vi "PC_RealTimeHardwareDetection.vi"() -> ()   [LabVIEW 2010]
uses:
  <vilib>/nisyscfg/Initialize (Control).vi
  <vilib>/nisyscfg/Close (System).vi
  <vilib>/nisyscfg/Close (Hardware).vi
  C:/Program Files (x86)/National Instruments/LabVIEW 2010/resource/objmgr/nisysapi.rc
  <vilib>/nisyscfg/nisyscfg.lvlib
panel:
  out "Experts":T1(array[cluster])
  in  "Target (localhost)":refnum<k21>="localhost"
  out "Results":string[][](table)
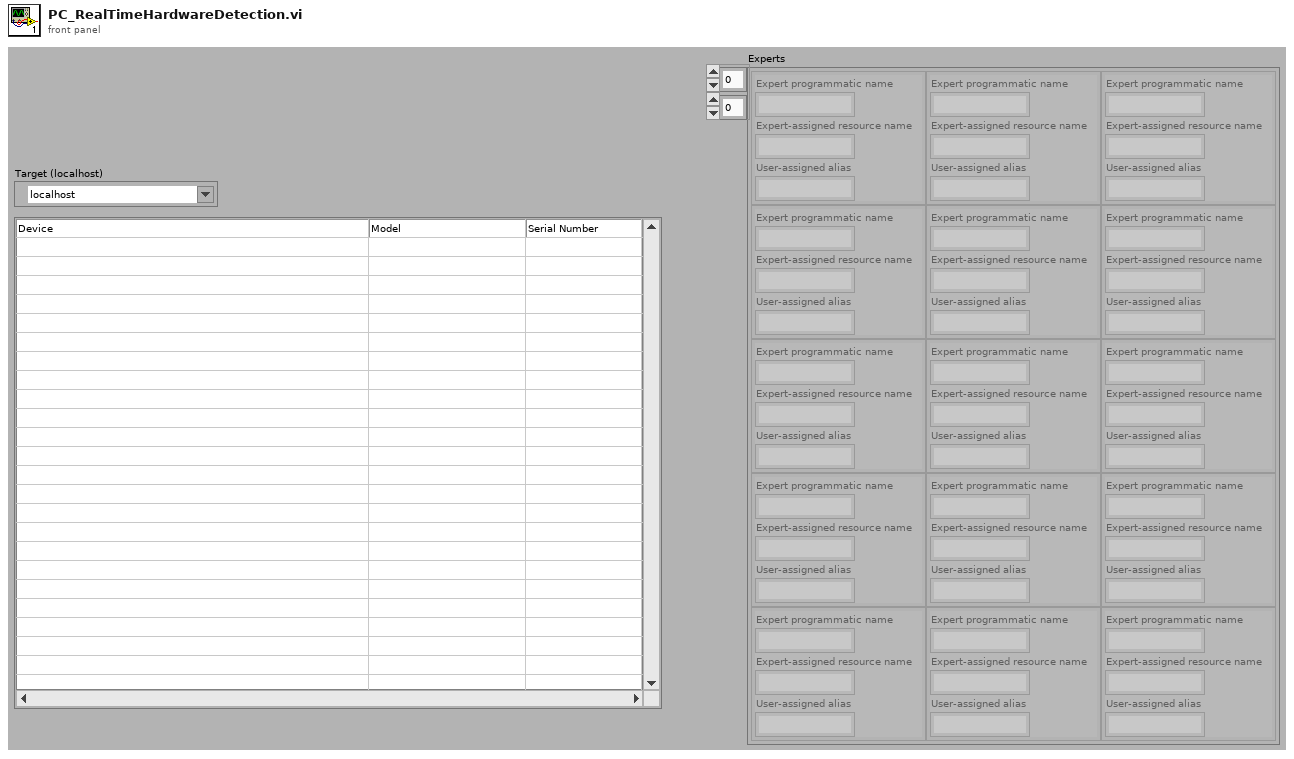
[diagram p1: front panel]
types:
  T1 = cluster{"Expert programmatic name":string, "Expert-assigned resource name":string, "User-assigned alias":string}[][]
  T2 = cluster{"Expert programmatic name":string, "Expert-assigned resource name":string, "User-assigned alias":string}[]
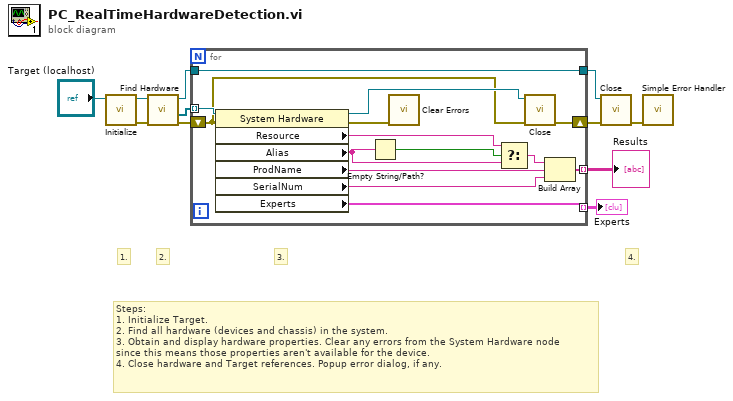
[diagram p0: block diagram]
diagram:
  # "4."
  # "3."
  # "2."
  # "1."
  # "Steps:\n1. Initialize Target.\n2. Find all hardware (devices and chassis) in the system.\n3. Obtain and display hardware properties. Clear any errors from the System Hardware node\nsince this means those properties aren't available for the device. \n4. Close hardware and Target references. Popup error dialog, if any."
  n1 = call-poly <vilib>:"Initialize.vi"("session in"="Target (localhost)") -> ("error out"=w10:errorcluster, "session out"=w11:refnum<k21>)  [unwired: 8 in, 1 out]
  n2 = call <vilib>:"Find Hardware.vi"("error in (no error)"=w10, "session in"=w11) -> ("error out"=w7:errorcluster, "resources out"=w8:refnum<k20>[], "session out"=w9:refnum<k21>)  [unwired: 1 in, 6 out]
  n3 = for {
    tunnel: [w25] -> w6
    tunnel: w9 -> [w25]
    tunnel: w8 -> [w22] mode=indexing
    shift-right: [w24] -> w5
    shift-left: w7 -> [w13]
    tunnel: [w16] -> w2 mode=indexing
    tunnel: [w12] -> w1 mode=indexing
    n4 = property class="System Hardware"(reference=w22, error in=w13) -> (reference out=w14:refnum<k20>, error out=w15:errorcluster, "Resource"=w20:string, "Alias"=w21:string, "ProdName"=w18:string, "SerialNum"=w17:string, "Experts"=w12:T2)
    n5 = Empty String/Path?(string/path=w21) -> (empty?=w23:bool)
    n6 = call <vilib>:"Clear Errors.vi"("error in (no error)"=w15) -> ()  [unwired: 6 in, 1 out]
    n7 = Select(t=w20, s=w23, f=w21) -> (s? t:f=w19:string)
    n8 = call-poly <vilib>:"Close.vi"("error in (no error)"=w13, "resource in"=w14) -> ("error out"=w24:errorcluster)  [unwired: 9 in]
    n9 = Build Array(w19, w18, w17) -> (w16:string[])
  }
  "Results" <- w2
  "Experts" <- w1
  n10 = call-poly <vilib>:"Close.vi"("error in (no error)"=w5, "session in"=w6) -> ("error out"=w4:errorcluster)  [unwired: 9 in]
  n11 = call <vilib>:"Simple Error Handler.vi"("error in (no error)"=w4) -> ()  [unwired: 4 in, 5 out]
